vi "PopUp_Select Language.vi"(8 "error in (no error)":errorcluster, 10 "Languages":T1[](array[typedef])) -> (0 "error out":errorcluster, 2 "OK Pressed?":bool, 3 "LangIndex":i32)   [LabVIEW 2013, in "SET Project Editor.lvlib"]
uses:
  SET Project Editor.lvlib
  SET Project Data/Types/ProjFile_Language Entry.ctl
  DialogEnum.ctl
  SET Project Data/SET Project Data.lvlib
panel:
  in  "Language":i32(ring) items=["English", "French"]
  in  "Cancel":bool
  in  "OK":bool
  # "Select Language"
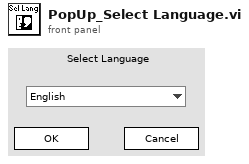
[diagram p1: front panel]
types:
  T1 = typedef "SET Project Data.lvlib/ProjFile_Language Entry.ctl" = cluster{"Tag":string, "Name":string, "Code Page":u16}
  T2 = typedef "SET Project Editor.lvlib/DialogEnum.ctl" = enum16{"Idle", "Init", "Shutdown"}
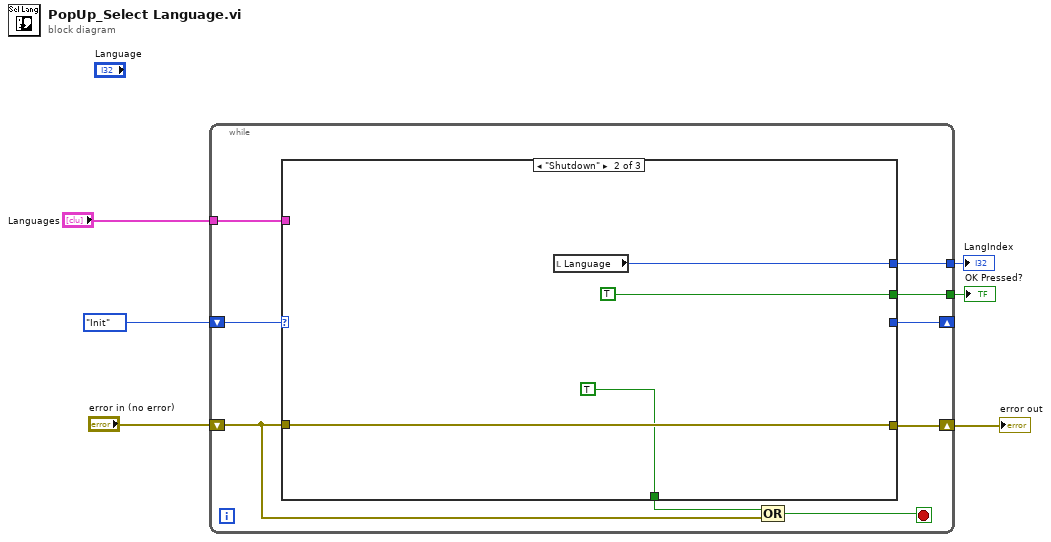
[diagram p0: block diagram]
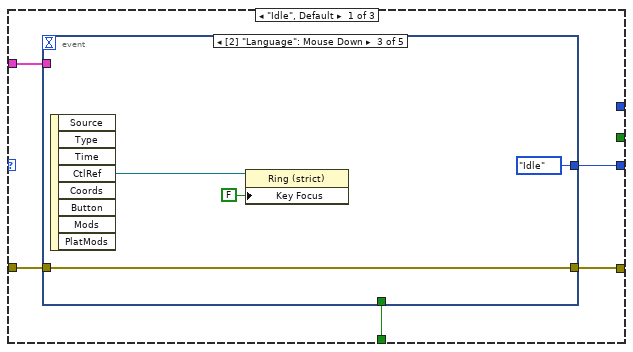
[diagram p2: hidden frame]
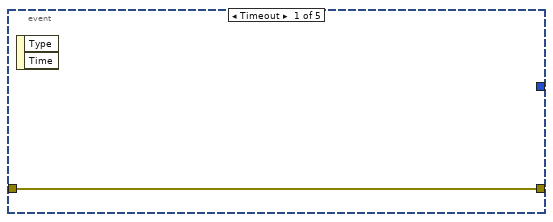
[diagram p3: hidden frame]
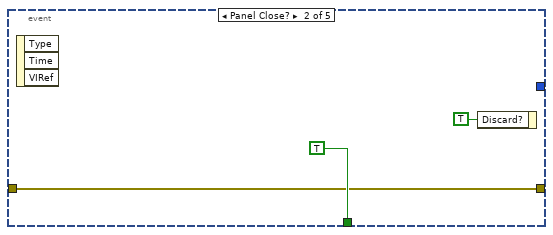
[diagram p4: hidden frame]
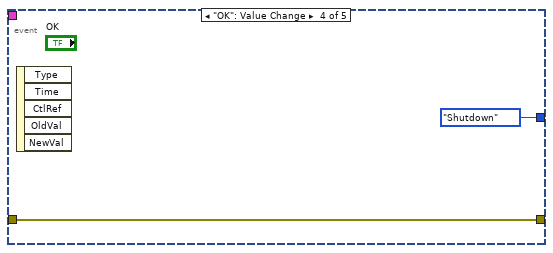
[diagram p5: hidden frame]
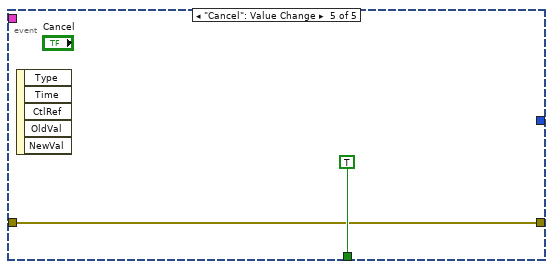
[diagram p6: hidden frame]
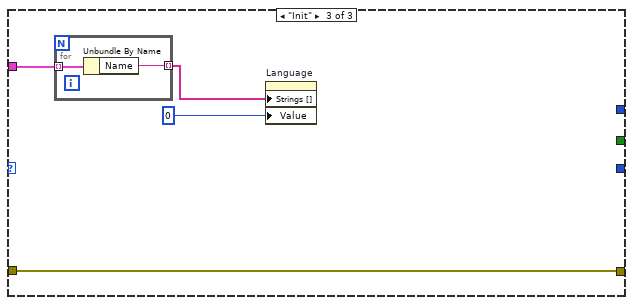
[diagram p7: hidden frame]
diagram:
  n1 = while {
    shift-right: [w14] -> w4
    shift-left: "error in (no error)" -> [w8]
    shift-right: [w13] -> _
    shift-left: DialogEnum."Init" -> [w15]
    tunnel: "Languages" -> [w12]
    tunnel: [w11] -> w3
    tunnel: [w10] -> w2
    stop <- w7 stop-if-true
    n2 = case shown="\"Shutdown\"" w15 {
      tunnel: [w20 w36 w40] -> w14
      tunnel: w8 -> [w19 w36 w40]
      tunnel: [w18 TRUE _] -> w9
      tunnel: [w17 _ _] -> w13
      tunnel: w12 -> [w16 _ w38]
      tunnel: [_ w34 _] -> w11
      tunnel: [_ TRUE _] -> w10
      frame "Idle", Default {
        n3 = event shown="[2] \"Language\": Mouse Down" {
          selector: _ -> [_ _ _ _ _]
          dyn-events: _ -> [_ _ _ _ _]
          timeout: _ -> [_ _ _ _ _]
          tunnel: [w21 w22 w26 w29 w31] -> w20
          tunnel: w19 -> [w21 w22 w26 w29 w31]
          tunnel: [_ TRUE _ _ TRUE] -> w18
          tunnel: [_ _ DialogEnum."Idle" DialogEnum."Shutdown" _] -> w17
          tunnel: w16 -> [_ _ _ _ _]
          event Timeout {
            n4 = event-data() -> ()  [unwired: 1 in, 2 out]
          }
          event Panel Close? {
            n5 = event-data() -> ()  [unwired: 1 in, 3 out]
            n6 = event-data("Discard?"=TRUE) -> ()  [unwired: 1 in, 1 out]
          }
          event "Language": Mouse Down {
            n7 = event-data() -> ("CtlRef"=w28:refnum<vi>)  [unwired: 1 in, 7 out]
            n8 = property class="Ring (strict)"(reference=w28, "Key Focus"=FALSE) -> ()  [unwired: 1 in, 2 out]
          }
          event "OK": Value Change {
            n9 = event-data() -> ()  [unwired: 1 in, 5 out]
          }
          event "Cancel": Value Change {
            n10 = event-data() -> ()  [unwired: 1 in, 5 out]
          }
        }
      }
      frame "Shutdown" {
        n11 = local read "Language"() -> (w34:i32)
      }
      frame "Init" {
        n12 = for {
          tunnel: w38 -> [w42] mode=indexing
          tunnel: [w41] -> w37 mode=indexing
          n13 = Unbundle By Name(w42) -> ("Name"=w41:string)
        }
        n14 = property on="Language" class="Ring (strict)"("Strings []"=w37, "Value"=0) -> ()  [unwired: 2 in, 2 out]
      }
    }
    n15 = Compound Arithmetic op=OR(w9, w8) -> (w7:bool)
  }
  "error out" <- w4
  "LangIndex" <- w3
  "OK Pressed?" <- w2
